vi "final.vi"() -> ()   [LabVIEW 2019]
uses:
  Program Files (x86)/National Instruments/LabVIEW 2019/project/EN1Course-master (12)/EN1Course-master/_Subs/SystemLink/SL_Subs/SL_XControl.xctl
  Program Files (x86)/National Instruments/LabVIEW 2019/project/EN1Course-master (12)/EN1Course-master/_Subs/SystemLink/SL_Subs/SystemLink_Write_String.vi
panel:
  in  "completion 2":T1(xcontrol)={"Tag"="Completed", "Type"="STRING", "Data"="Not Done Yet :("}
  in  "completion":T1(xcontrol)={"Tag"="Completed", "Type"="STRING", "Data"="Not Done Yet :("}
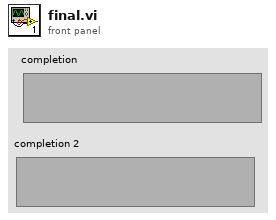
[diagram p1: front panel]
types:
  T1 = cluster{"Tag":string, "Type":string, "Data":string}
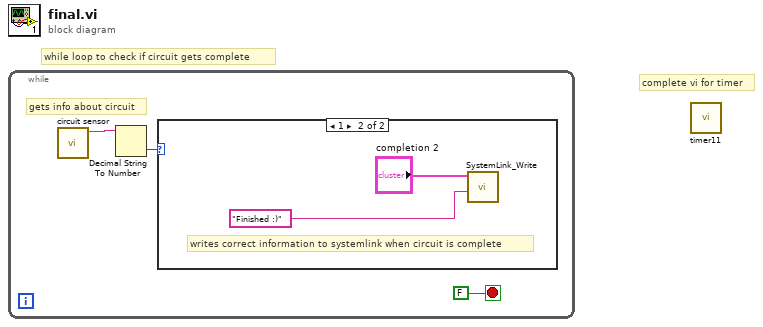
[diagram p0: block diagram]
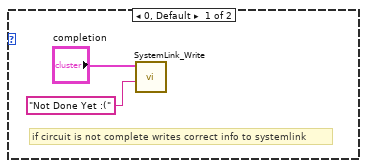
[diagram p2: hidden frame]
diagram:
  # "while loop to check if circuit gets complete"
  # "complete vi for timer"
  n1 = while {
    stop <- FALSE stop-if-true
    # "gets info about circuit"
    n2 = call "circuit sensor.vi"() -> ("Property (str)"=w3:string)  [unwired: 11 in]
    n3 = Decimal String To Number(string=w3) -> (number=w2:i32)  [unwired: 2 in, 1 out]
    n4 = case shown="1" w2 {
      frame 0, Default {
        # "if circuit is not complete writes correct info to systemlink"
        n5 = call-poly "SystemLink_Write.vi"("String"="Not Done Yet :(", "SL_XControl"="completion") -> ()  [unwired: 10 in]
      }
      frame 1 {
        # "writes correct information to systemlink when circuit is complete"
        n6 = call-poly "SystemLink_Write.vi"("String"="Finished :)", "SL_XControl"="completion 2") -> ()  [unwired: 10 in]
      }
    }
  }
  n7 = call "timer11.vi"() -> ()  [unwired: 12 in]
